vi "Is CSM Module.vi"(8 "error in (no error)":errorcluster, 11 "VIRef":refnum<vi>) -> (0 "error out":errorcluster, 2 "Is CSM Module?":bool, 3 "VIRef(dup)":refnum<vi>)   [LabVIEW 2017, in "CSM-Helper.lvclass"]
uses:
  CSM-Helper.lvclass
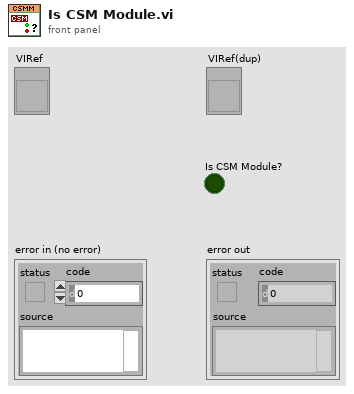
[diagram p1: front panel]
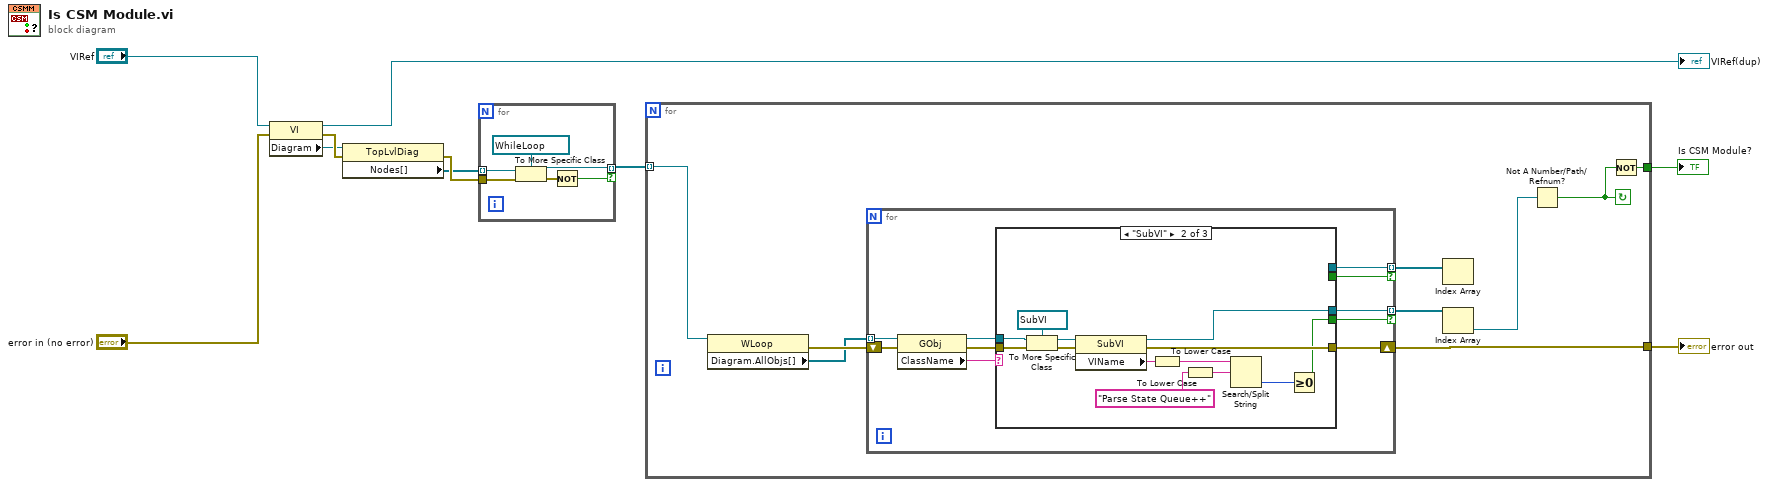
[diagram p0: block diagram]
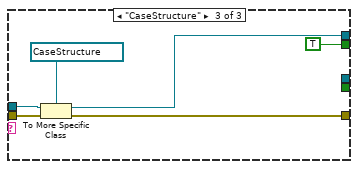
[diagram p3: hidden frame]
diagram:
  n1 = property on="Property Node" class="VI"(reference="VIRef", error in="error in (no error)") -> (reference out=→"VIRef(dup)":refnum<vi>, error out=w8:errorcluster, "Diagram"=w5:refnum<vi>)
  n2 = property on="Property Node" class="TopLvlDiag"(reference=w5, error in=w8) -> (error out=w7:errorcluster, "Nodes[]"=w6:refnum<vi>[])  [unwired: 1 out]
  n3 = for {
    tunnel: w6 -> [w15] mode=indexing
    tunnel: [w13] -> w4 mode=indexing if=w11
    tunnel: w7 -> [w14]
    n4 = To More Specific Class(target class=refnum<vi> refnum ("WLoop Refnum"), reference=w15, error in=w14) -> (specific class reference=w13:refnum<vi>, error out=w12:errorcluster)
    n5 = Not(x=w12) -> (.not. x?=w11:bool)
  }
  n6 = for {
    tunnel: w4 -> [w24] mode=indexing
    tunnel: [w25] -> w3
    tunnel: [w21] -> w1
    stop <- w22 continue-if-true
    n7 = property on="Property Node" class="WLoop"(reference=w24) -> (error out=w18:errorcluster, "Diagram.AllObjs[]"=w17:refnum<vi>[])  [unwired: 1 in, 1 out]
    n8 = for {
      tunnel: w17 -> [w35] mode=indexing
      shift-right: [w30] -> w25
      shift-left: w18 -> [w31]
      tunnel: [w29] -> w20 mode=indexing if=w26
      tunnel: [w28] -> w19 mode=indexing if=w27
      n9 = property class="GObj"(reference=w35, error in=w31) -> (reference out=w33:refnum<vi>, error out=w32:errorcluster, "ClassName"=w34:string)
      n10 = case shown="\"SubVI\"" w34 {
        tunnel: w33 -> [_ w48 w54]
        tunnel: w32 -> [w36 w47 w53]
        tunnel: [w36 w42 w52] -> w30
        tunnel: [_ w41 _] -> w29
        tunnel: [_ _ w51] -> w28
        tunnel: [_ _ TRUE] -> w27
        tunnel: [_ w37 _] -> w26
        frame Default {
        }
        frame "SubVI" {
          n11 = To More Specific Class(target class=refnum<vi> refnum ("SubVI Refnum"), reference=w48, error in=w47) -> (specific class reference=w46:refnum<vi>, error out=w45:errorcluster)
          n12 = property class="SubVI"(reference=w46, error in=w45) -> (reference out=w41:refnum<vi>, error out=w42:errorcluster, "VIName"=w44:string)
          n13 = To Lower Case(string=w44) -> (all lower case string=w39:string)
          n14 = To Lower Case(string="Parse State Queue++" ("VI Name")) -> (all lower case string=w40:string)
          n15 = Search/Split String(string=w39, search string/char (-)=w40) -> (offset of match=w38:i32)  [unwired: 1 in, 2 out]
          n16 = Greater Or Equal To 0?(x=w38) -> (x >= 0?=w37:bool)
        }
        frame "CaseStructure" {
          n17 = To More Specific Class(target class=refnum<vi> refnum ("CaseSel Refnum"), reference=w54, error in=w53) -> (specific class reference=w51:refnum<vi>, error out=w52:errorcluster)
        }
      }
    }
    n18 = Index Array(array=w19) -> ()  [unwired: 1 in, 1 out]
    n19 = Index Array(array=w20) -> (element=w23:refnum<vi>)  [unwired: 1 in]
    n20 = Not A Number/Path/Refnum?(number/path/refnum=w23) -> (NaN/Path/Refnum?=w22:bool)
    n21 = Not(x=w22) -> (.not. x?=w21:bool)
  }
  "error out" <- w3
  "Is CSM Module?" <- w1
